vi "VS-Test HR From EKG.vi"(0 "Cluster In":T2) -> (4 "Cluster out":T2)   [LabVIEW 2020]
uses:
  Typedefs/PhysMon-HR From EKG Settings.ctl
  epl-vi-lib/Utility VIs/Buttons/KCheckmarkBoolean 2.ctl
panel:
  in  "Save waveform":T1
  out "Heart Rate (bpm)":dbl format="%.1f"
  in  "Acquire":bool
  out "XY Graph":cluster{"Array":dbl[], "Filtered X":dbl[]}[](graph)
  in  "Finished":bool
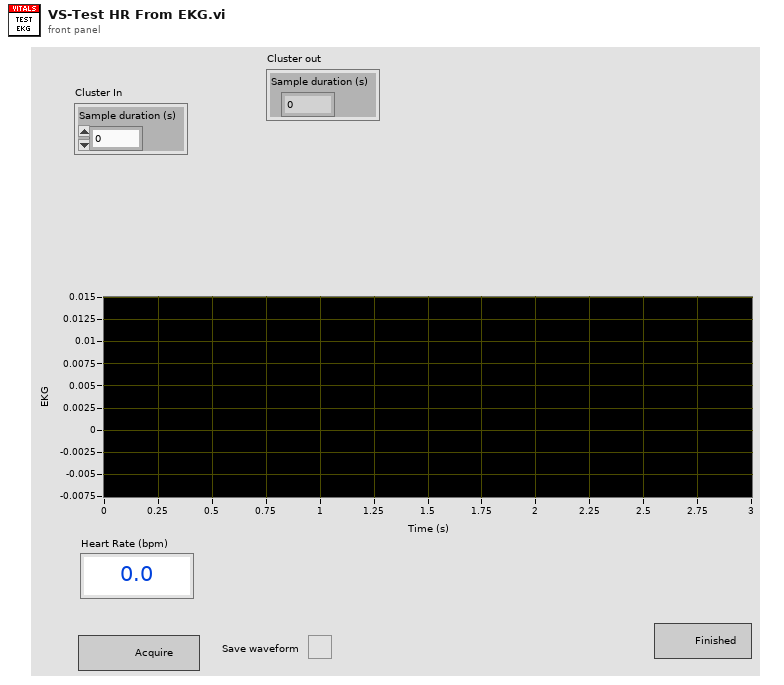
[diagram p1: front panel]
types:
  T1 = typedef "KCheckmarkBoolean 2.ctl" = bool
  T2 = typedef "PhysMon-HR From EKG Settings.ctl" = cluster{"Sample duration (s)":dbl}
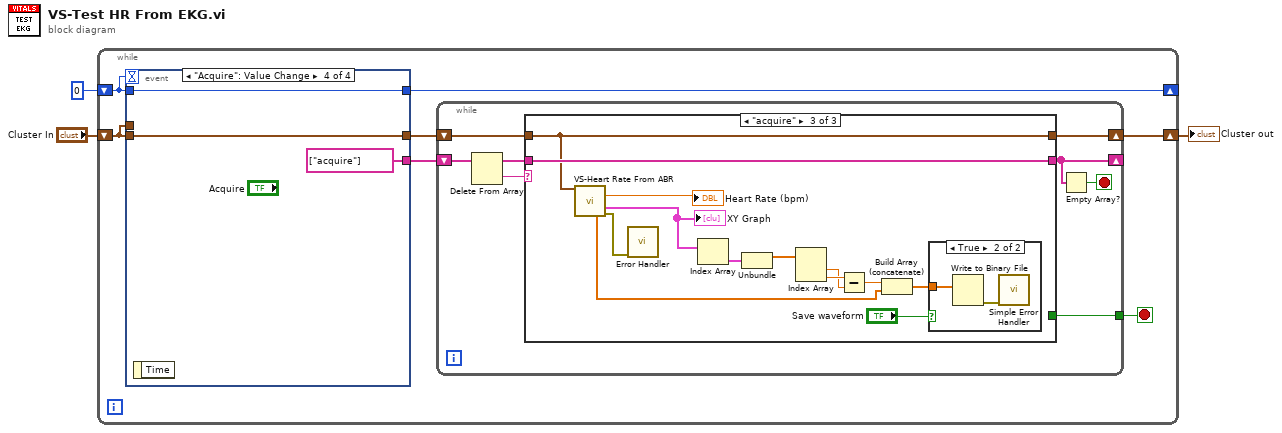
[diagram p0: block diagram]
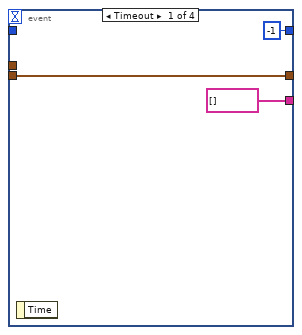
[diagram p2: hidden frame]
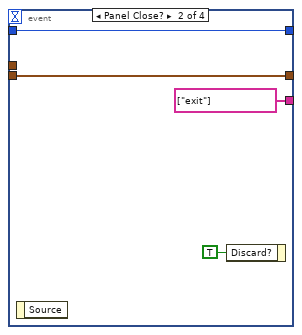
[diagram p3: hidden frame]
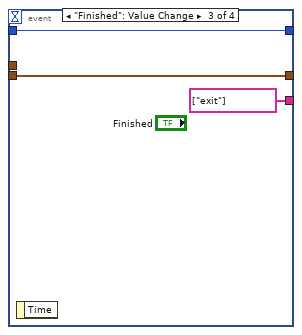
[diagram p4: hidden frame]
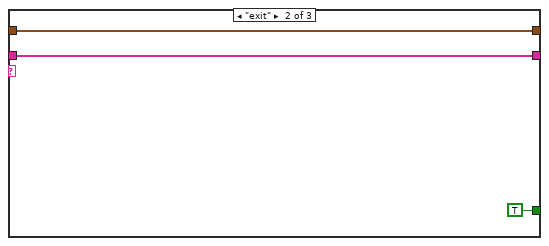
[diagram p6: hidden frame]
diagram:
  n1 = while {
    shift-right: [w10] -> _
    shift-left: 0 -> [w8]
    shift-right: [w4] -> w1
    shift-left: "Cluster In" -> [w9]
    stop <- w5 stop-if-true
    n2 = event shown="[3] \"Acquire\": Value Change" {
      selector: _ -> [_ _ _ _]
      dyn-events: _ -> [_ _ _ _]
      timeout: w8 -> [_ _ _ _]
      tunnel: [-1 w17 w20 w23] -> w10
      tunnel: w9 -> [w12 w16 w18 w21]
      tunnel: [w12 w16 w18 w21] -> w7
      tunnel: w9 -> [_ _ _ _]
      tunnel: w8 -> [_ w17 w20 w23]
      tunnel: [string[] [] string[] ["exit"] string[] ["exit"] string[] ["acquire"]] -> w6
      event Timeout {
        n3 = event-data() -> ()  [unwired: 1 in, 1 out]
      }
      event Panel Close? {
        n4 = event-data() -> ()  [unwired: 1 in, 1 out]
        n5 = event-data("Discard?"=TRUE) -> ()  [unwired: 1 in, 1 out]
      }
      event "Finished": Value Change {
        n6 = event-data() -> ()  [unwired: 1 in, 1 out]
      }
      event "Acquire": Value Change {
        n7 = event-data() -> ()  [unwired: 1 in, 1 out]
      }
    }
    n8 = while {
      shift-right: [w28] -> _
      shift-left: w6 -> [w31]
      shift-right: [w25] -> w4
      shift-left: w7 -> [w26]
      tunnel: [w24] -> w5
      stop <- w27 stop-if-true
      n9 = Delete From Array(array=w31) -> (deleted portion=w29:string, array with subset deleted=w30:string[])  [unwired: 2 in]
      n10 = case shown="\"acquire\"" w29 {
        tunnel: w30 -> [w33 w36 w49]
        tunnel: [w33 w36 w49] -> w28
        tunnel: w26 -> [w32 w35 w48]
        tunnel: [w32 w35 w48] -> w25
        tunnel: [_ TRUE _] -> w24
        frame "", Default {
        }
        frame "exit" {
        }
        frame "acquire" {
          n11 = call "VS-Heart Rate From ABR.vi"("Settings"=w48) -> ("Heart Rate (bpm)"=→"Heart Rate (bpm)":dbl, "XY Graph"=w45:cluster{"Array":dbl[], "Filtered X":dbl[]}[], "Raw waveform"=w37:dbl[], "error out"=w46:errorcluster)  [unwired: 11 in]
          "XY Graph" <- w45
          n12 = call "Error Handler.vi"("error in (no error)"=w46) -> ()  [unwired: 13 in, 2 out]
          n13 = Index Array(array=w45) -> (element=w44:cluster{"Array":dbl[], "Filtered X":dbl[]})  [unwired: 1 in]
          n14 = Unbundle(w44) -> ("Array"=w42:dbl[])  [unwired: 1 out]
          n15 = Index Array(array=w42) -> (element #1=w40:dbl, element #2=w41:dbl)  [unwired: 2 in]
          n16 = Subtract(x=w41, y=w40) -> (x-y=w39:dbl)
          n17 = Build Array (concatenate)(w39, w37) -> (w38:dbl[])
          n18 = case shown="True" "Save waveform" {
            tunnel: w38 -> [_ w51]
            frame False {
            }
            frame True {
              n19 = Write to Binary File(data=w51) -> (error out=w50:errorcluster)  [unwired: 5 in, 2 out]
              n20 = call <vilib>:"Simple Error Handler.vi"("error in (no error)"=w50) -> ()  [unwired: 4 in, 5 out]
            }
          }
        }
      }
      n21 = Empty Array?(array=w28) -> (empty?=w27:bool)
    }
  }
  "Cluster out" <- w1
